vi "Set Window Position (left, top).vi"(0 "VI in":refnum<vi>, 7 "Coords":T1) -> (4 "VI out":refnum<vi>, 15 "error out":errorcluster)   [LabVIEW 2020]
uses:
  <vilib>/Utility/miscctls.llb/LVPoint32TypeDef.ctl
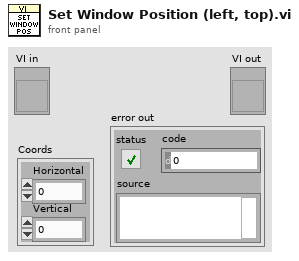
[diagram p1: front panel]
types:
  T1 = typedef "LVPoint32TypeDef.ctl" = cluster{"Horizontal":i32, "Vertical":i32}
  T2 = typedef "LVRectTypeDef.ctl" = cluster{"Left":i16, "Top":i16, "Right":i16, "Bottom":i16}
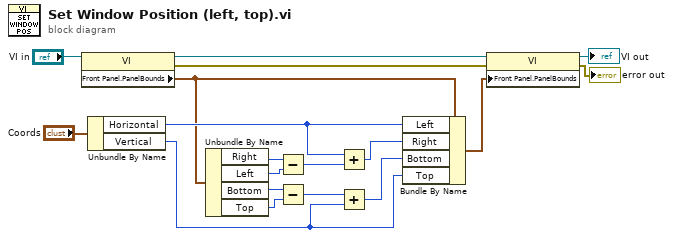
[diagram p0: block diagram]
diagram:
  n1 = property class="VI"(reference="VI in") -> (reference out=w5:refnum<vi>, error out=w7:errorcluster, "Front Panel.PanelBounds"=w16:T2)  [unwired: 1 in]
  n2 = Unbundle By Name("Coords") -> ("Horizontal"=w18:i32, "Vertical"=w17:i32)
  n3 = Unbundle By Name(w16) -> ("Right"=w3:i16, "Left"=w14:i16, "Bottom"=w4:i16, "Top"=w15:i16)
  n4 = Subtract(x=w3, y=w14) -> (x-y=w8:i16)
  n5 = Subtract(x=w4, y=w15) -> (x-y=w9:i16)
  n6 = Add(x=w18, y=w8) -> (x+y=w10:i32)
  n7 = Add(x=w9, y=w17) -> (x+y=w11:i32)
  n8 = Bundle By Name(cluster=w16, "Left"=w18, "Right"=w10, "Bottom"=w11, "Top"=w17) -> (w12:T2)
  n9 = property class="VI"(reference=w5, error in=w7, "Front Panel.PanelBounds"=w12) -> (reference out=→"VI out":refnum<vi>, error out=→"error out":errorcluster)
